vi "RollingDice-NoSubVI.vi"() -> ()   [LabVIEW 2019]
panel:
  out "You Win":bool
  out "You Lose":bool
  out "Sum":dbl
  in  "Roll Dice":bool
  out "Dice 2":dbl
  out "Dice 1":dbl
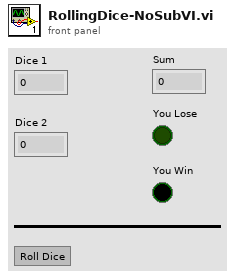
[diagram p1: front panel]
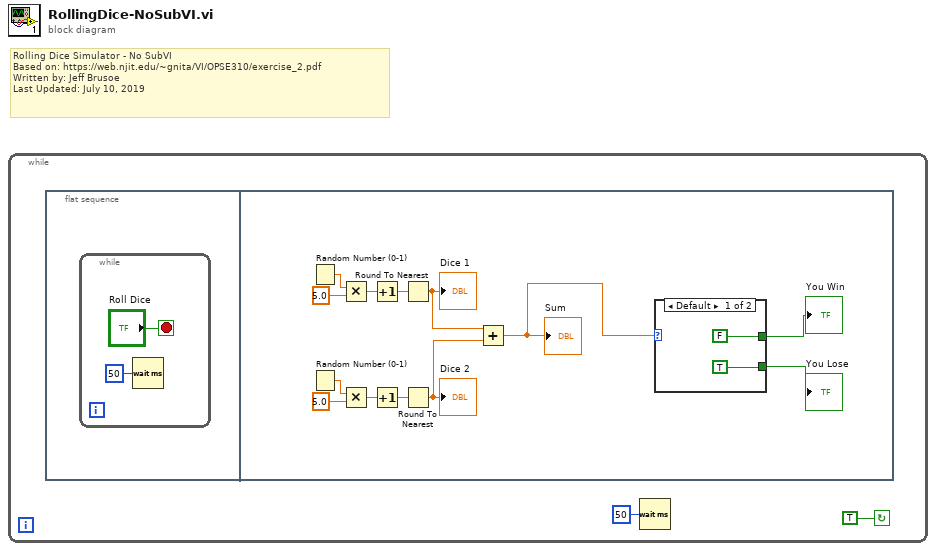
[diagram p0: block diagram]
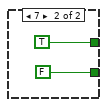
[diagram p2: hidden frame]
diagram:
  # "Rolling Dice Simulator - No SubVI\nBased on: https://web.njit.edu/~gnita/VI/OPSE310/exercise_2.pdf\nWritten by: Jeff Brusoe\nLast Updated: July 10, 2019"
  n1 = while {
    stop <- TRUE continue-if-true
    n2 = flat-sequence {
      frame #0 {
        n3 = while {
          stop <- "Roll Dice" stop-if-true
          n4 = Wait (ms)(milliseconds to wait=u32 50) -> ()  [unwired: 1 out]
        }
      }
      frame #1 {
        n5 = Random Number (0-1)() -> (number: 0 to 1=w12:dbl)
        n6 = Random Number (0-1)() -> (number: 0 to 1=w15:dbl)
        n7 = Multiply(x=w12, y=5.0) -> (x*y=w13:dbl)
        n8 = Multiply(x=w15, y=5.0) -> (x*y=w16:dbl)
        n9 = Increment(x=w13) -> (x+1=w14:dbl)
        n10 = Increment(x=w16) -> (x+1=w17:dbl)
        n11 = Round To Nearest(number=w14) -> (nearest integer value=w9:dbl)
        "Dice 1" <- w9
        n12 = Round To Nearest(number=w17) -> (nearest integer value=w8:dbl)
        "Dice 2" <- w8
        n13 = Add(x=w9, y=w8) -> (x+y=w7:dbl)
        "Sum" <- w7
        n14 = case shown="Default" w7 {
          tunnel: [FALSE TRUE] -> w6
          tunnel: [TRUE FALSE] -> w5
          frame Default {
          }
          frame 7 {
          }
        }
        "You Win" <- w6
        "You Lose" <- w5
      }
    }
    n15 = Wait (ms)(milliseconds to wait=u32 50) -> ()  [unwired: 1 out]
  }
